vi "XYGraphOptions.vi"(4 "Plot.Plot Interpolation":u8, 6 "Plot.Point Style":u8, 7 "Numeric Control":i32, 9 "Plot.Line Width":u8, 10 "Plot.Line Style":u8, 11 "XYGraph in":refnum<vi>) -> (3 "Array":u32[](array[numeric]))   [LabVIEW 2014]
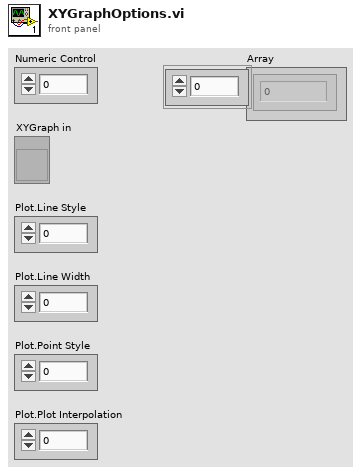
[diagram p1: front panel]
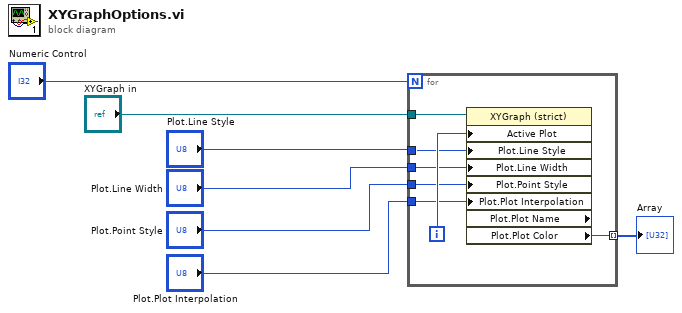
[diagram p0: block diagram]
diagram:
  n1 = for {
    N: "Numeric Control" -> [_]
    tunnel: "XYGraph in" -> [w14]
    tunnel: "Plot.Line Style" -> [w12]
    tunnel: "Plot.Line Width" -> [w11]
    tunnel: "Plot.Point Style" -> [w10]
    tunnel: "Plot.Plot Interpolation" -> [w9]
    tunnel: [w8] -> w7 mode=indexing
    i -> [w13]
    n2 = property class="XYGraph (strict)" props=["Active Plot", "Plot", "Line Style", "Plot", "Line Width", "Plot", "Point Style", "Plot", "Plot Interpolation", "Plot", "Plot Name", "Plot", "Plot Color"](reference=w14, "Active Plot"=w13, "Plot.Line Style"=w12, "Plot.Line Width"=w11, "Plot.Point Style"=w10, "Plot.Plot Interpolation"=w9) -> ("Plot.Plot Color"=w8:u32)  [unwired: 1 in, 3 out]
  }
  "Array" <- w7
